vi "DM_Control_Main_V3.vi"() -> ()   [LabVIEW 2014]
uses:
  Controls/Pixel Scan Parameters.ctl
  Controls/MirrorModes.ctl
  Controls/Standard Action.ctl
  <vilib>/Analysis/baseanly.llb/Mean (DBL).vi
  <vilib>/Utility/file.llb/Write To Spreadsheet File (DBL).vi
  <vilib>/Utility/file.llb/Read From Spreadsheet File (DBL).vi
  <vilib>/Analysis/NI_AALBase.lvlib
panel:
  in  "Choose DM":u16(ring) items=["isoSTED Upper", "isoSTED Lower"]
  in  "Load Flat":bool
  in  "Apply Zero":bool
  in  "Load V Map":bool
  in  "Save V Map":bool
  in  "Apply Flat":bool
  in  "Center Bias":bool
  in  "Exit":bool
  in  "Mirror Tab":enum32{"Mirror Modes", "Scan Pixels"}(tab)
  in  "Clear Modes":bool
  in  "Mirror Modes":T1
  in  "Load Modes":bool
  in  "Save Modes":bool
  in  "Scan Modes":bool
  in  "Pixel Scan Parameters":T2={"Scan Start Pixel"=1, "Scan End Pixel"=1, "Pixel Start Value (-1 to 1)"=-0.5, "Pixel End Value (-1 to 1)"=0.5, "Number of Steps"=0.1}
  in  "Start Pixel Scan":bool
  out "Pixel Map (-1 to 1)":dbl[][](graph)
  # "Mode"
  # "Amount (nm)"
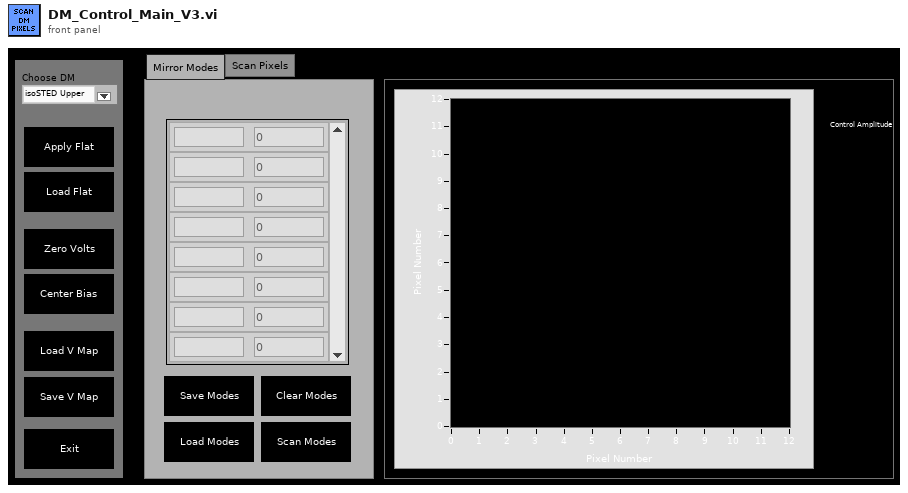
[diagram p1: front panel]
types:
  T1 = typedef "MirrorModes.ctl" = cluster{"Mode":string, "Amplitude":dbl}[]
  T2 = typedef "Pixel Scan Parameters.ctl" = cluster{"Scan Start Pixel":i32, "Scan End Pixel":i32, "Pixel Start Value (-1 to 1)":dbl, "Pixel End Value (-1 to 1)":dbl, "Number of Steps":dbl}
  T3 = typedef "Standard Action.ctl" = enum16{"Read", "Write"}
  T4 = enum16{"Start Scan", "Reset Counter", "Write DM", "Get Image", "Update Count", "Exit"}
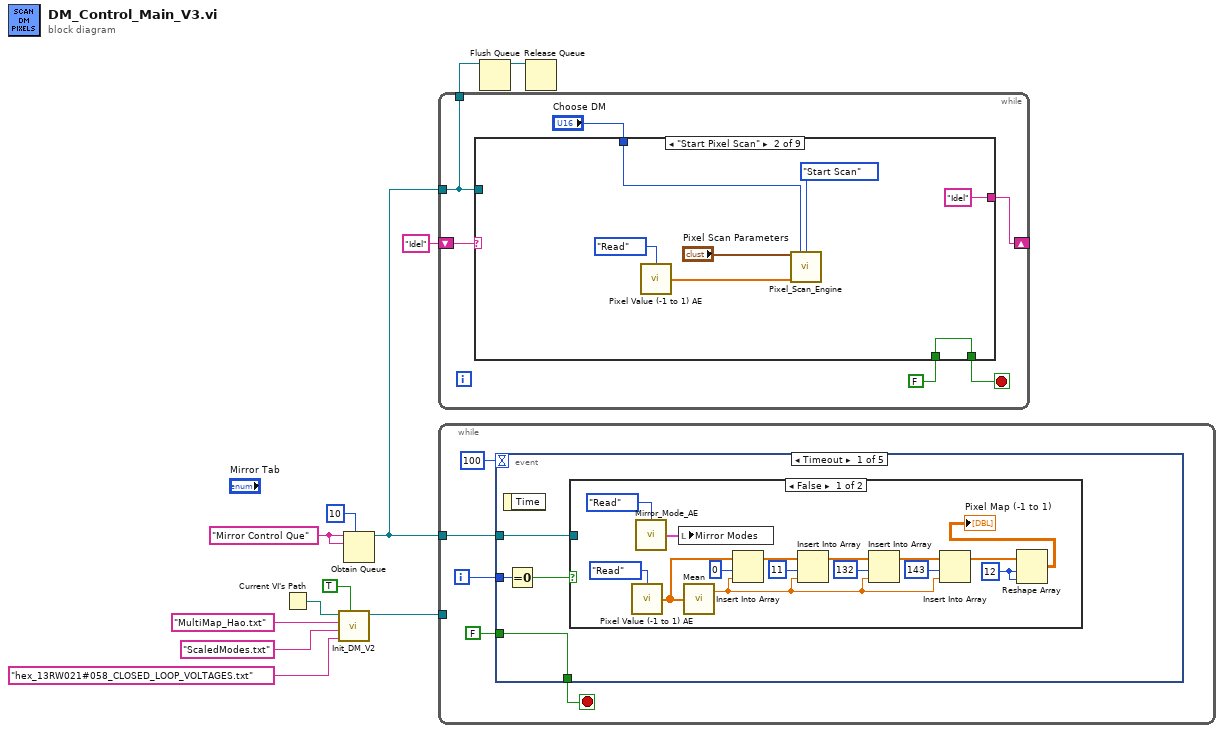
[diagram p0: block diagram]
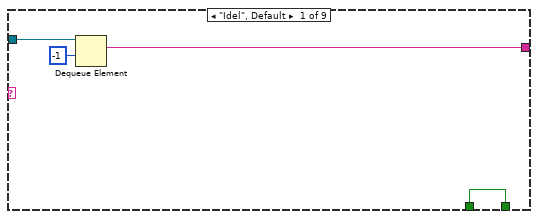
[diagram p2: hidden frame]
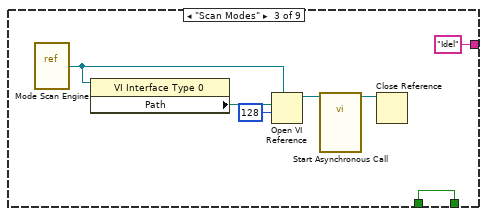
[diagram p3: hidden frame]
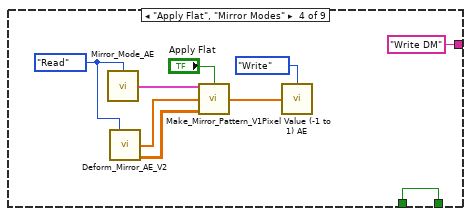
[diagram p4: hidden frame]
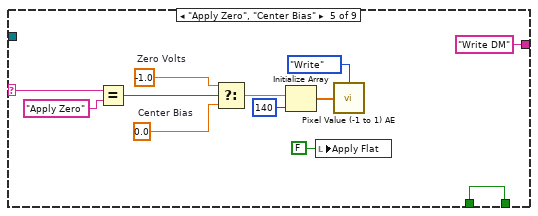
[diagram p5: hidden frame]
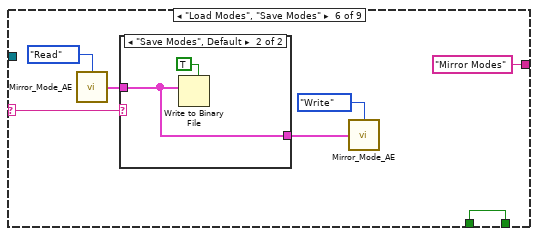
[diagram p6: hidden frame]
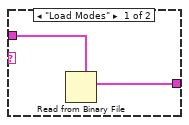
[diagram p7: hidden frame]
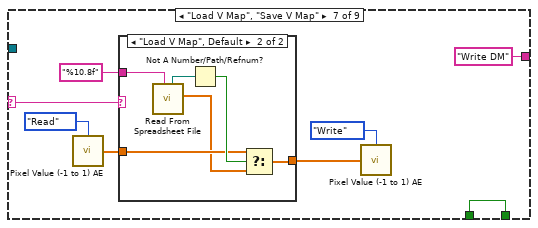
[diagram p8: hidden frame]
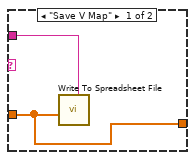
[diagram p9: hidden frame]
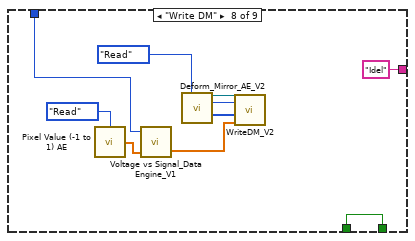
[diagram p10: hidden frame]
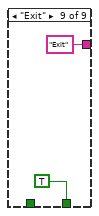
[diagram p11: hidden frame]
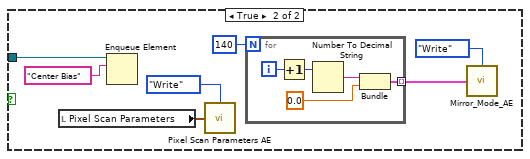
[diagram p12: hidden frame]
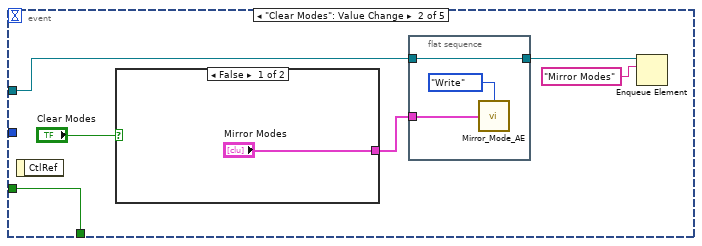
[diagram p13: hidden frame]
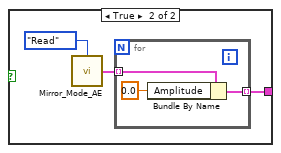
[diagram p14: hidden frame]
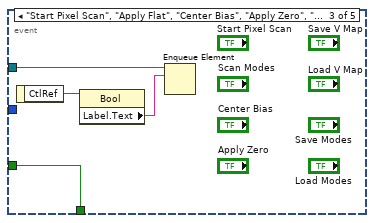
[diagram p15: hidden frame]
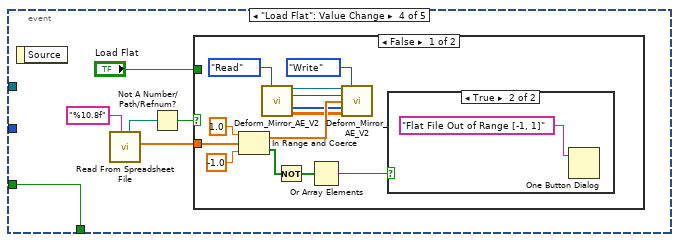
[diagram p16: hidden frame]
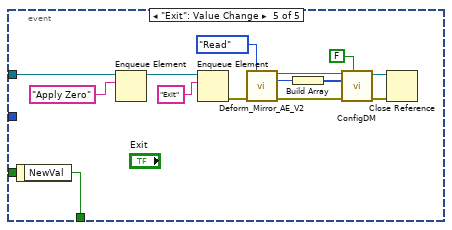
[diagram p19: hidden frame]
diagram:
  w12 = "Mirror Control Que" ("name (unnamed)")
  n1 = Current VI's Path() -> (path=w4:path)
  n2 = call "Init_DM_V2.vi"("BM Flat"=TRUE, "BM Flat File"="hex_13RW021#058_CLOSED_LOOP_VOLTAGES.txt" ("name or relative path"), "Mirror Modes File"="ScaledModes.txt" ("name or relative path"), "DM Mapping File"="MultiMap_Hao.txt" ("name or relative path"), "Base File Path"=w4) -> ("reference out"=w10:refnum<k7>)  [unwired: 6 in]
  n3 = Obtain Queue(max queue size (-1, unlimited)=10, name (unnamed)=w12, element data type=w12) -> (queue out=w6:refnum<queue>)  [unwired: 2 in, 2 out]
  n4 = while {
    tunnel: w6 -> [w14]
    shift-right: [w18] -> _
    shift-left: "Idel" ("name (unnamed)") -> [w17]
    tunnel: [w14] -> w9
    stop <- w16 stop-if-true
    n5 = case shown="\"Start Pixel Scan\"" w17 {
      selector: w17 -> [_ _ _ _ w52 w60 w75 _ _]
      tunnel: w14 -> [w22 _ _ _ _ _ _ _ _]
      tunnel: [w20 "Idel" ("name (unnamed)") "Idel" ("name (unnamed)") "Write DM" ("name (unnamed)") "Write DM" ("name (unnamed)") "Mirror Modes" ("name (unnamed)") "Write DM" ("name (unnamed)") "Idel" ("name (unnamed)") "Exit" ("name (unnamed)")] -> w18
      tunnel: [w19 w29 w36 w44 w57 w64 w76 w94 TRUE] -> w16
      tunnel: FALSE -> [w19 w29 w36 w44 w57 w64 w76 w94 _]
      tunnel: "Choose DM" -> [_ w23 _ _ _ _ _ w86 _]
      frame "Idel", Default {
        n6 = Dequeue Element(queue=w22, timeout in ms (-1)=-1) -> (element=w20:string)  [unwired: 1 in, 3 out]
      }
      frame "Start Pixel Scan" {
        n7 = call "Pixel Value (-1 to 1) AE.vi"("Action"=Standard_Action."Read") -> ("Pixel Value (-1 to 1) Out"=w27:dbl[])  [unwired: 14 in]
        n8 = call "Pixel_Scan_Engine.vi"("Pixel Scan Parameters In"="Pixel Scan Parameters", "DM #"=w23, "Action"=T4."Start Scan", "Initial Pixel Values (-1 to 1)"=w27) -> ()  [unwired: 12 in]
      }
      frame "Scan Modes" {
        n9 = vi-ref "Mode Scan Engine.vi"() -> (w30:refnum<vi>)
        n10 = property class="VI Interface Type 0"(reference=w30) -> ("Path"=w31:path)  [unwired: 1 in, 2 out]
        n11 = Open VI Reference(type specifier VI Refnum (for type only)=w30, vi path=w31, options=128) -> (vi reference=w33:refnum<vi>)  [unwired: 3 in, 1 out]
        n12 = call-by-ref "Start Asynchronous Call"(reference=w33) -> (reference out=w34:refnum<vi>)  [unwired: 17 in, 1 out]
        n13 = Close Reference(reference=w34) -> ()  [unwired: 1 in, 1 out]
      }
      frame "Apply Flat", "Mirror Modes" {
        w38 = Standard_Action."Read" ("Action")
        n14 = call "Mirror_Mode_AE.vi"("Action"=w38) -> ("Mirror Modes Out"=w41:T1)  [unwired: 14 in]
        n15 = call "Deform_Mirror_AE_V2.vi"("Action"=w38) -> ("Flat Files Out"=w42:dbl[], "Mode Matrix Out"=w43:dbl[][])  [unwired: 10 in, 3 out]
        n16 = call "Make_Mirror_Pattern_V1.vi"("Mirror Modes In"=w41, "Flat On?"="Apply Flat", "Flat File In"=w42, "Mirror Modes Array"=w43) -> ("Pixel Value U (-1 to 1)"=w40:dbl[])  [unwired: 11 in]
        n17 = call "Pixel Value (-1 to 1) AE.vi"("Action"=Standard_Action."Write", "Pixel Value (-1 to 1)"=w40) -> ()  [unwired: 13 in, 1 out]
      }
      frame "Apply Zero", "Center Bias" {
        w48 = -1.0  # Zero Volts
        w50 = 0.0  # Center Bias
        n18 = Equal?(x=w52, y="Apply Zero") -> (x = y?=w51:bool)
        n19 = Select(t=w48, s=w51, f=w50) -> (s? t:f=w49:dbl)
        n20 = Initialize Array(w49, 140 ("dimension size")) -> (w55:dbl[])
        n21 = local write "Apply Flat"(FALSE ("Apply Flat")) -> ()
        n22 = call "Pixel Value (-1 to 1) AE.vi"("Action"=Standard_Action."Write", "Pixel Value (-1 to 1)"=w55) -> ()  [unwired: 13 in, 1 out]
      }
      frame "Load Modes", "Save Modes" {
        n23 = call "Mirror_Mode_AE.vi"("Action"=Standard_Action."Read") -> ("Mirror Modes Out"=w59:T1)  [unwired: 14 in]
        n24 = case shown="\"Save Modes\", Default" w60 {
          tunnel: w59 -> [w66 w67]
          tunnel: [w65 w67] -> w58
          frame "Load Modes" {
            n25 = Read from Binary File(5:w66) -> (2:w65:T1)  [unwired: 5 in, 3 out]
          }
          frame "Save Modes", Default {
            n26 = Write to Binary File(data=w67, 5:TRUE ("prepend array or string size? (T)")) -> ()  [unwired: 4 in, 3 out]
          }
        }
        n27 = call "Mirror_Mode_AE.vi"("Action"=Standard_Action."Write", "Mirror Modes In"=w58) -> ()  [unwired: 13 in, 1 out]
      }
      frame "Load V Map", "Save V Map" {
        n28 = call "Pixel Value (-1 to 1) AE.vi"("Action"=Standard_Action."Read") -> ("Pixel Value (-1 to 1) Out"=w73:dbl[])  [unwired: 14 in]
        n29 = case shown="\"Load V Map\", Default" w75 {
          tunnel: w73 -> [w77 w81]
          tunnel: "%10.8f" -> [w78 w84]
          tunnel: [w77 w79] -> w69
          frame "Save V Map" {
            n30 = call-poly <vilib>:"Write To Spreadsheet File.vi"("format (%.3f)"=w78, "1D data"=w77) -> ()  [unwired: 6 in, 1 out]
          }
          frame "Load V Map", Default {
            n31 = call-poly <vilib>:"Read From Spreadsheet File.vi"("format (%.3f)"=w84) -> ("first row"=w80:dbl[], "new file path (Not A Path if cancelled)"=w83:path)  [unwired: 6 in, 3 out]
            n32 = Not A Number/Path/Refnum?(number/path/refnum=w83) -> (NaN/Path/Refnum?=w82:bool)
            n33 = Select(t=w81, s=w82, f=w80) -> (s? t:f=w79:dbl[])
          }
        }
        n34 = call "Pixel Value (-1 to 1) AE.vi"("Action"=Standard_Action."Write", "Pixel Value (-1 to 1)"=w69) -> ()  [unwired: 13 in, 1 out]
      }
      frame "Write DM" {
        n35 = call "Pixel Value (-1 to 1) AE.vi"("Action"=Standard_Action."Read") -> ("Pixel Value (-1 to 1) Out"=w87:dbl[])  [unwired: 14 in]
        n36 = call "Voltage vs Signal_Data Engine_V1.vi"("Control Signal In (-1~1)"=w87, "DM #"=w86) -> ("Voltage Out (0~Max. Vol.)"=w88:dbl[])  [unwired: 1 in, 1 out]
        n37 = call "Deform_Mirror_AE_V2.vi"("Action"=Standard_Action."Read") -> ("Refnum Out"=w91:refnum<k7>, "IDs Out"=w90:i32, "Multi Map Data Out"=w89:i32[])  [unwired: 10 in, 2 out]
        n38 = call "WriteDM_V2.vi"("reference in"=w91, "nDevId"=w90, "MultiDM  Mapping"=w89, "Voltage Array in"=w88) -> ()  [unwired: 2 in, 2 out]
      }
      frame "Exit" {
      }
    }
  }
  n39 = while {
    tunnel: w6 -> [w97]
    tunnel: w10 -> [_]
    i -> [w98]
    stop <- w101 stop-if-true
    n40 = event shown="[0] Timeout" {
      selector: _ -> [_ _ _ _ _]
      dyn-events: _ -> [_ _ _ _ _]
      timeout: 100 -> [_ _ _ _ _]
      tunnel: [w105 w138 w152 w158 w185] -> w101
      tunnel: FALSE -> [w105 w138 w152 w158 _]
      tunnel: w98 -> [w104 _ _ _ _]
      tunnel: w97 -> [w102 w137 w151 _ w183]
      event Timeout {
        n41 = event-data() -> ()  [unwired: 1 in, 1 out]
        n42 = Equal To 0?(x=w104) -> (x = 0?=w103:bool)
        n43 = case shown="False" w103 {
          tunnel: w102 -> [_ w127]
          frame False {
            w119 = 12 ("dimension size")
            n44 = call "Pixel Value (-1 to 1) AE.vi"("Action"=Standard_Action."Read") -> ("Pixel Value (-1 to 1) Out"=w120:dbl[])  [unwired: 14 in]
            n45 = call "Mirror_Mode_AE.vi"("Action"=Standard_Action."Read") -> ("Mirror Modes Out"=w107:T1)  [unwired: 14 in]
            n46 = local write "Mirror Modes"(w107) -> ()
            n47 = call-poly <vilib>:"Mean.vi"("X"=w120) -> ("mean"=w117:dbl)  [unwired: 1 out]
            n48 = Insert Into Array(array=w120, index=0, new element=w117) -> (w112:dbl[])
            n49 = Insert Into Array(array=w112, index=11, new element=w117) -> (w114:dbl[])
            n50 = Insert Into Array(array=w114, index=132, new element=w117) -> (w116:dbl[])
            n51 = Insert Into Array(array=w116, index=143, new element=w117) -> (w109:dbl[])
            n52 = Reshape Array(w109, w119, w119) -> (→"Pixel Map (-1 to 1)":dbl[][])
          }
          frame True {
            n53 = local read "Pixel Scan Parameters"() -> (w124:T2)
            n54 = Enqueue Element(queue=w127, element="Center Bias") -> ()  [unwired: 2 in, 3 out]
            n55 = call "Pixel Scan Parameters AE.vi"("Action"=enum16{"Write", "Read"}."Write", "Pixel Scan Parameters"=w124) -> ()  [unwired: 13 in, 1 out]
            n56 = for {
              N: 140 -> [_]
              tunnel: [w128] -> w121 mode=indexing
              i -> [w132]
              n57 = Increment(x=w132) -> (x+1=w131:i32)
              n58 = Number To Decimal String(number=w131) -> (decimal integer string=w130:string)  [unwired: 1 in]
              n59 = Bundle(w130, 0.0) -> (w128:cluster{string, dbl})  [unwired: 1 in]
            }
            n60 = call "Mirror_Mode_AE.vi"("Action"=Standard_Action."Write", "Mirror Modes In"=w121) -> ()  [unwired: 13 in, 1 out]
          }
        }
      }
      event "Clear Modes": Value Change {
        n61 = event-data() -> ()  [unwired: 1 in, 1 out]
        n62 = case shown="False" "Clear Modes" {
          tunnel: ["Mirror Modes" w140] -> w133
          frame False {
          }
          frame True {
            n63 = call "Mirror_Mode_AE.vi"("Action"=Standard_Action."Read") -> ("Mirror Modes Out"=w142:T1)  [unwired: 14 in]
            n64 = for {
              tunnel: w142 -> [w145] mode=indexing
              tunnel: [w143] -> w140 mode=indexing
              n65 = Bundle By Name(cluster=w145, "Amplitude"=0.0) -> (w143:cluster{"Mode":string, "Amplitude":dbl})
            }
          }
        }
        n66 = flat-sequence {
          tunnel: w133 -> [w147]
          tunnel: w137 -> [w146]
          tunnel: [w146] -> w135
          frame #0 {
            n67 = call "Mirror_Mode_AE.vi"("Action"=Standard_Action."Write", "Mirror Modes In"=w147) -> ()  [unwired: 13 in, 1 out]
          }
        }
        n68 = Enqueue Element(queue=w135, element="Mirror Modes") -> ()  [unwired: 2 in, 3 out]
      }
      event "Start Pixel Scan", "Apply Flat", "Center Bias", "Apply Zero", "Save V Map", "Save Modes", "Load Modes", "Load V Map", "Scan Modes": Value Change {
        n69 = event-data() -> ("CtlRef"=w150:refnum<vi>)  [unwired: 1 in]
        n70 = property class="Bool"(reference=w150) -> ("Label.Text"=w149:string)  [unwired: 1 in, 2 out]
        n71 = Enqueue Element(queue=w151, element=w149) -> ()  [unwired: 2 in, 3 out]
      }
      event "Load Flat": Value Change {
        n72 = event-data() -> ()  [unwired: 1 in, 1 out]
        n73 = call-poly <vilib>:"Read From Spreadsheet File.vi"("format (%.3f)"="%10.8f") -> ("first row"=w154:dbl[], "new file path (Not A Path if cancelled)"=w156:path)  [unwired: 6 in, 3 out]
        n74 = Not A Number/Path/Refnum?(number/path/refnum=w156) -> (NaN/Path/Refnum?=w155:bool)
        n75 = case shown="False" w155 {
          tunnel: w154 -> [w171 _]
          tunnel: "Load Flat" -> [_ _]
          frame False {
            n76 = In Range and Coerce(upper limit=1.0, x=w171, lower limit=-1.0) -> (coerced(x)=w164:dbl[], In Range?=w168:bool[])
            n77 = call "Deform_Mirror_AE_V2.vi"("Action"=Standard_Action."Read") -> ("Refnum Out"=w160:refnum<k7>, "IDs Out"=w161:i32, "Multi Map Data Out"=w162:i32[], "Mode Matrix Out"=w163:dbl[][])  [unwired: 10 in, 1 out]
            n78 = Not(x=w168) -> (.not. x?=w167:bool[])
            n79 = Or Array Elements(Boolean array=w167) -> (logical OR=w159:bool)
            n80 = call "Deform_Mirror_AE_V2.vi"("Refnum In"=w160, "Action"=Standard_Action."Write", "IDs In"=w161, "Flat Files In"=w164, "Multi Map Data In"=w162, "Mode Matrix"=w163) -> ()  [unwired: 5 in, 5 out]
            n81 = case shown="True" w159 {
              frame False {
              }
              frame True {
                n82 = One Button Dialog(message="Flat File Out of Range [-1, 1]") -> ()  [unwired: 1 in, 1 out]
              }
            }
          }
          frame True {
          }
        }
      }
      event "Exit": Value Change {
        n83 = event-data() -> ("NewVal"=w185:bool)  [unwired: 1 in]
        n84 = Enqueue Element(queue=w183, element="Apply Zero") -> (queue out=w182:refnum<queue>)  [unwired: 2 in, 2 out]
        n85 = Enqueue Element(queue=w182, element="Exit") -> (error out=w174:errorcluster)  [unwired: 2 in, 2 out]
        n86 = call "Deform_Mirror_AE_V2.vi"("Action"=Standard_Action."Read") -> ("Refnum Out"=w177:refnum<k7>, "IDs Out"=w178:i32)  [unwired: 10 in, 3 out]
        n87 = Build Array(w178) -> (w179:i32[])
        n88 = call "ConfigDM.vi"("High Voltage"=FALSE, "error in (no error)"=w174, "Dev IDs"=w179, "Automation Refnum in"=w177) -> ("error out"=w173:errorcluster, "Automation Refnum out"=w176:refnum<k7>)  [unwired: 6 in]
        n89 = Close Reference(reference=w176, error in (no error)=w173) -> ()  [unwired: 1 out]
      }
    }
  }
  n90 = Flush Queue(queue=w9) -> (queue out=w8:refnum<queue>)  [unwired: 1 in, 2 out]
  n91 = Release Queue(queue=w8) -> ()  [unwired: 2 in, 3 out]
